vi "Configure Chassis Identity.vi"(8 "error in (no error)":errorcluster, 10 "Chassis Identity (0)":i32, 11 "Chassis VISA resource name":refnum<visa-resource-name>) -> (0 "error out":errorcluster, 3 "Chassis VISA resource name out":refnum<visa-resource-name>)   [LabVIEW 2018, in "Agilent U2722.lvlib"]
doc: "This VI sets the Chassis's Identity number.\n\n<B>Note: </B>\nThe VISA resouce name of this VI should be the 2781 chassis' VISA resource name."
uses:
  Agilent U2722.lvlib
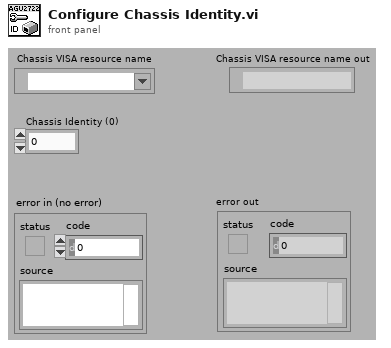
[diagram p1: front panel]
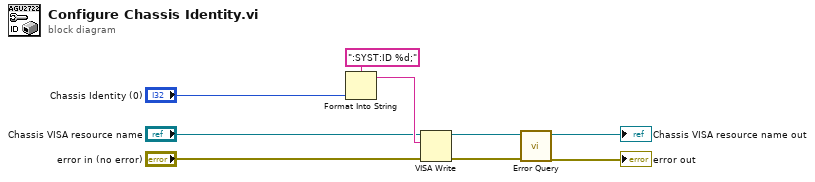
[diagram p0: block diagram]
diagram:
  n1 = Format Into String(format string=":SYST:ID %d;", "Chassis Identity (0)") -> (resulting string=w7:string)  [unwired: 2 in, 1 out]
  n2 = VISA Write(VISA resource name="Chassis VISA resource name", write buffer=w7, error in (no error)="error in (no error)") -> (VISA resource name out=w4:refnum<visa-resource-name>, error out=w3:errorcluster)  [unwired: 1 out]
  n3 = call "Error Query.vi"("error in (no error)"=w3, "VISA resource name"=w4) -> ("error out"=→"error out":errorcluster, "VISA resource name out"=→"Chassis VISA resource name out":refnum<visa-resource-name>)  [unwired: 6 in, 2 out]
